vi "LHF.DB.Mongo.Client.Connect.vi"(8 "error in (no error)":errorcluster, 9 "database":string, 10 "url":string, 11 "LHF.DB.Mongo in":refnum<class "LHF.DB.Mongo.lvclass">) -> (0 "error out":errorcluster, 3 "LHF.DB.Mongo out":refnum<class "LHF.DB.Mongo.lvclass">)   [LabVIEW 2013, in "LHF.DB.Mongo.lvclass"]
doc: "url format:\nmongodb://[username:password@]host1[:port1][,host2[:port2],...[,hostN[:portN]]][/[database][?options]]"
uses:
  LHF.DB.Mongo.lvclass
  C:/Users/Ricardo/Desktop/Projetos/LabVIEW-MongoDB/src/Driver/MongoDB.Driver.dll
  LabVIEW-MongoDB/src/Driver/MongoDB.Driver.dll
  LHF.DB.Mongo.lvclass/LHF.DB.Mongo.ctl
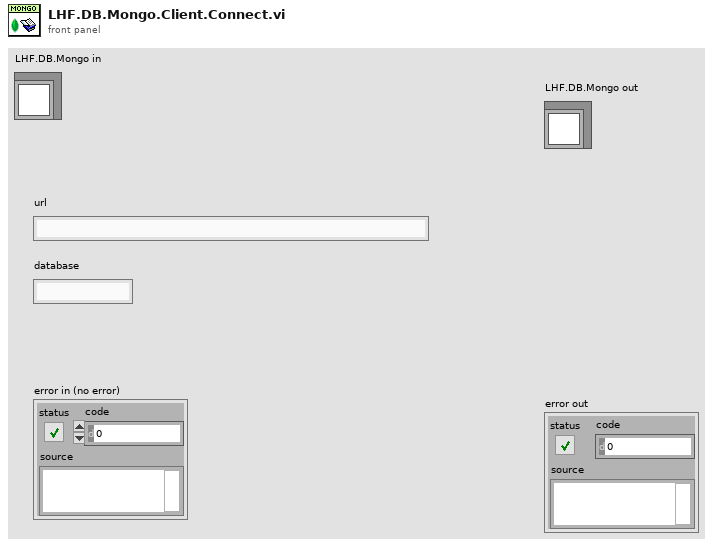
[diagram p1: front panel]
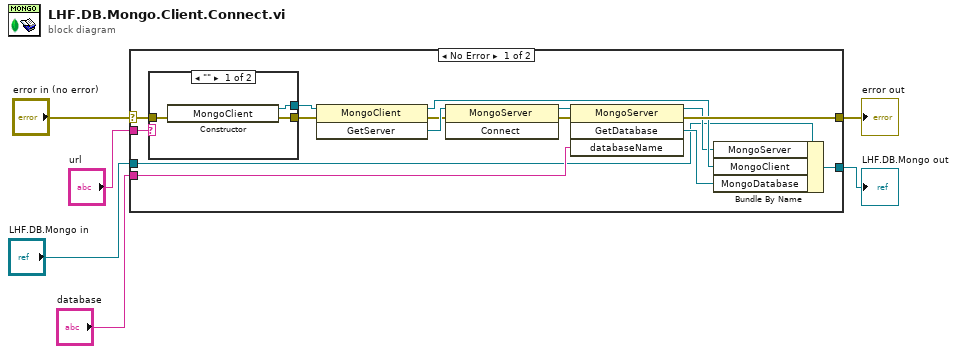
[diagram p0: block diagram]
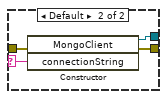
[diagram p2: hidden frame]
diagram:
  n1 = case shown="No Error" "error in (no error)" {
    selector: "error in (no error)" -> [w8 w30]
    tunnel: "url" -> [w7 _]
    tunnel: "database" -> [w18 _]
    tunnel: [w17 w30] -> w3
    tunnel: "LHF.DB.Mongo in" -> [w9 w29]
    tunnel: [w15 w29] -> w1
    frame No Error {
      n2 = case shown="\"\"" w7 {
        selector: w7 -> [_ w25]
        tunnel: [w24 w28] -> w21
        tunnel: [w23 w27] -> w19
        tunnel: w8 -> [w22 w26]
        frame "" {
          n3 = constructor class="MongoClient"(error in=w22) -> (reference out=w24:refnum<k24>, error out=w23:errorcluster)  [unwired: 2 in, 1 out]
        }
        frame Default {
          n4 = constructor class="MongoClient"(error in=w26, "connectionString"=w25) -> (reference out=w28:refnum<k24>, error out=w27:errorcluster)  [unwired: 2 in, 2 out]
        }
      }
      n5 = invoke class="MongoClient" method="GetServer"(reference=w21, error in=w19) -> (reference out=w16:refnum<k24>, error out=w12:errorcluster, "GetServer"=w20:refnum<k24>)  [unwired: 1 in]
      n6 = invoke class="MongoServer" method="Connect"(reference=w20, error in=w12) -> (reference out=w10:refnum<k24>, error out=w11:errorcluster)  [unwired: 1 in, 1 out]
      n7 = invoke class="MongoServer" method="GetDatabase"(reference=w10, error in=w11, "databaseName"=w18) -> (reference out=w14:refnum<k24>, error out=w17:errorcluster, "GetDatabase"=w13:refnum<k24>)  [unwired: 1 in, 1 out]
      n8 = Bundle By Name(cluster=w9, "MongoServer"=w14, "MongoClient"=w16, "MongoDatabase"=w13) -> (w15:refnum<class "LHF.DB.Mongo.lvclass">)
    }
    frame Error {
    }
  }
  "error out" <- w3
  "LHF.DB.Mongo out" <- w1
